vi "Launch Handler.vi"(6 "UUID":string, 8 "Super Data Model":refnum<class "Super Data Model.lvclass">, 9 "transmission data unit":refnum<class "Transmission Data Unit.lvclass">, 10 "connection reference":refnum<data-value>, 11 "TCP slave":refnum<class "TCP Slave.lvclass">) -> (0 "error out":errorcluster)   [LabVIEW 2013, in "Modbus Library - Advance.lvlib" / "TCP Slave.lvclass"]
doc: "Asynchronously launches a connection handler."
uses:
  TCP Slave.lvclass
  Transmission Data Unit/Transmission Data Unit.lvclass
  Super Data Model/Super Data Model.lvclass
  Connection.ctl
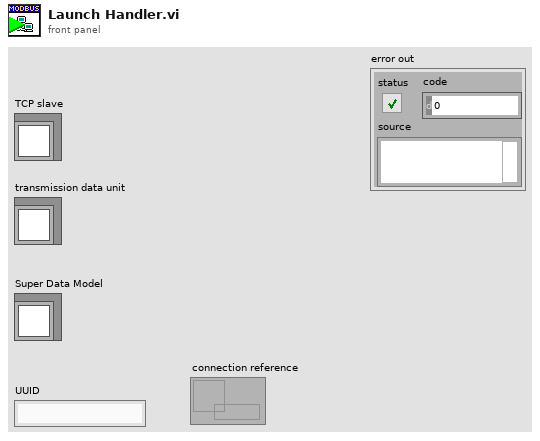
[diagram p1: front panel]
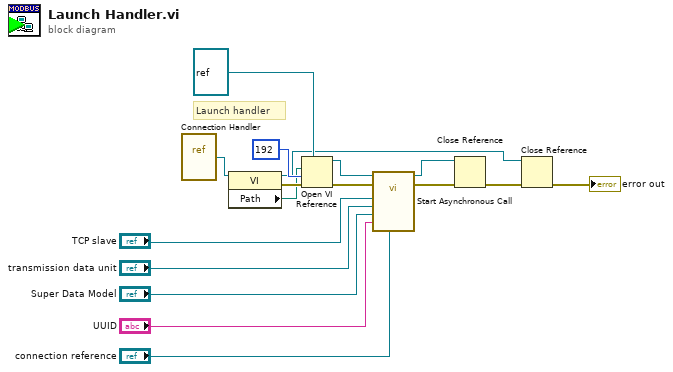
[diagram p0: block diagram]
diagram:
  # "Launch handler"
  n1 = vi-ref "Connection Handler.vi"() -> (w16:refnum<vi>)
  n2 = property class="VI"(reference=w16) -> (reference out=w1:refnum<vi>, error out=w15:errorcluster, "Path"=w13:path)  [unwired: 1 in]
  n3 = Open VI Reference(type specifier VI Refnum (for type only)=refnum<vi> refnum, vi path=w13, options=192 ("x .or. y?"), error in (no error)=w15) -> (vi reference=w10:refnum<vi>, error out=w11:errorcluster)  [unwired: 2 in]
  n4 = call-by-ref "Start Asynchronous Call"(reference=w10, error in=w11, "connection reference"="connection reference", "UUID"="UUID", "Super Data Model"="Super Data Model", "transmission data unit"="transmission data unit", "TCP slave"="TCP slave") -> (reference out=w2:refnum<vi>, error out=w5:errorcluster)  [unwired: 7 in]
  n5 = Close Reference(reference=w2, error in (no error)=w5) -> (error out=w4:errorcluster)
  n6 = Close Reference(reference=w1, error in (no error)=w4) -> (error out=→"error out":errorcluster)
